vi "settings_load_from_file.vi"(11 "XML File Path":path) -> (1 "Aux Data":string, 2 "Red Tweezers Version String":string)   [LabVIEW 2015]
uses:
  red_tweezers_globals_INTERNAL_VOLATILE.vi
  <vilib>/Utility/xml.llb/Read From XML File(array).vi
panel:
  out "VIs Loaded":string[](array[string])
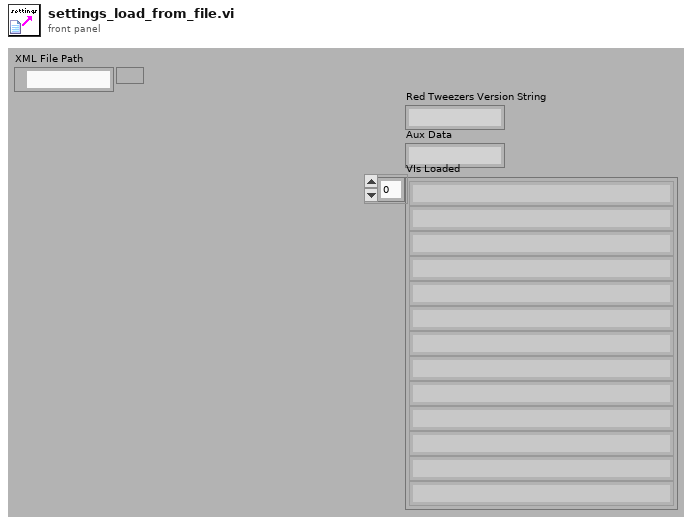
[diagram p1: front panel]
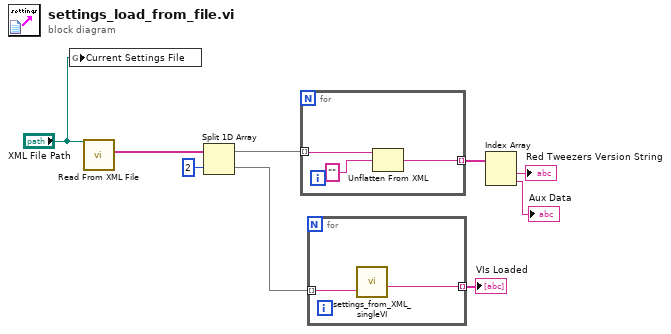
[diagram p0: block diagram]
diagram:
  n1 = global write "red_tweezers_globals_INTERNAL_VOLATILE.vi" "Current Settings File"("XML File Path") -> ()
  n2 = call-poly <vilib>:"Read From XML File.vi"("XML File Path"="XML File Path") -> ("XML Elements"=w8:string[])  [unwired: 8 in, 2 out]
  n3 = Split 1D Array(array=w8, index=2) -> (first subarray=w6:string[], second subarray=w9:string[])
  n4 = for {
    tunnel: w6 -> [w12] mode=indexing
    tunnel: [w10] -> w5 mode=indexing
    n5 = Unflatten From XML(xml string=w12, type="" ("XML in")) -> (value=w10:string)  [unwired: 1 in, 1 out]
  }
  n6 = for {
    tunnel: w9 -> [w14] mode=indexing
    tunnel: [w13] -> w2 mode=indexing
    n7 = call "settings_from_XML_singleVI.vi"("XML in"=w14) -> ("VI"=w13:string)  [unwired: 2 in, 2 out]
  }
  "VIs Loaded" <- w2
  n8 = Index Array(array=w5) -> (element #1=→"Red Tweezers Version String":string, element #2=→"Aux Data":string)  [unwired: 2 in]
